vi "Auto Transmission control.vi"(6 "Shift Constants":T1, 7 "In High Gear?":bool, 8 "Time of last recomended shift":u32, 9 "Is Turning?":bool, 10 "Commanded Throttle":dbl, 11 "Avg  encoder speed in fps":dbl) -> (0 "Time of last recomended shift":u32, 3 "should be High Gear?":bool)   [LabVIEW 2013]
uses:
  Shift Constants.ctl
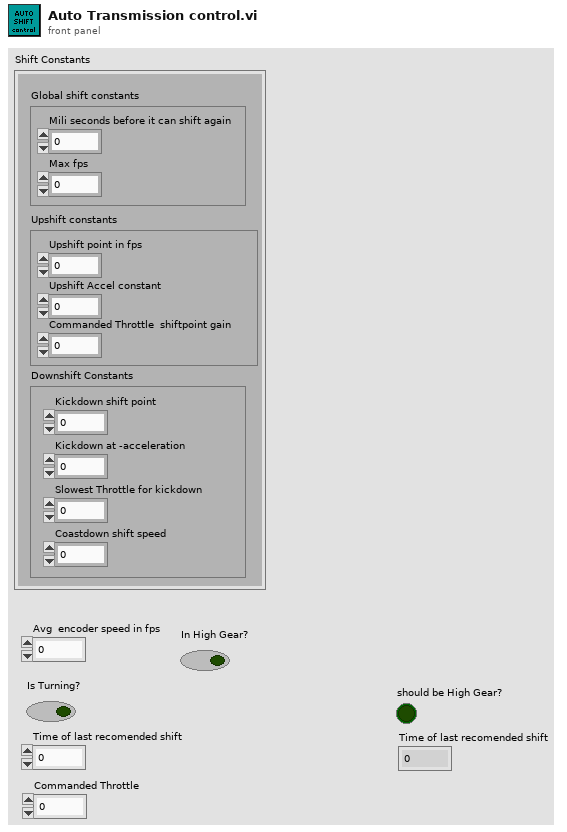
[diagram p1: front panel]
types:
  T1 = typedef "Shift Constants.ctl" = cluster{"Global shift constants":cluster{"Mili seconds before it can shift again":u32, "Max fps":dbl}, "Upshift constants":cluster{"Upshift point in fps":dbl, "Upshift Accel constant":dbl, "Commanded Throttle  shiftpoint gain":dbl}, "Downshift Constants":cluster{"Kickdown shift point":dbl, "Kickdown at -acceleration":dbl, "Slowest Throttle for kickdown":dbl, "Coastdown shift speed":dbl}}
  T2 = cluster{"Mili seconds before it can shift again":u32, "Max fps":dbl}
  T3 = cluster{"Upshift point in fps":dbl, "Upshift Accel constant":dbl, "Commanded Throttle  shiftpoint gain":dbl}
  T4 = cluster{"Kickdown shift point":dbl, "Kickdown at -acceleration":dbl, "Slowest Throttle for kickdown":dbl, "Coastdown shift speed":dbl}
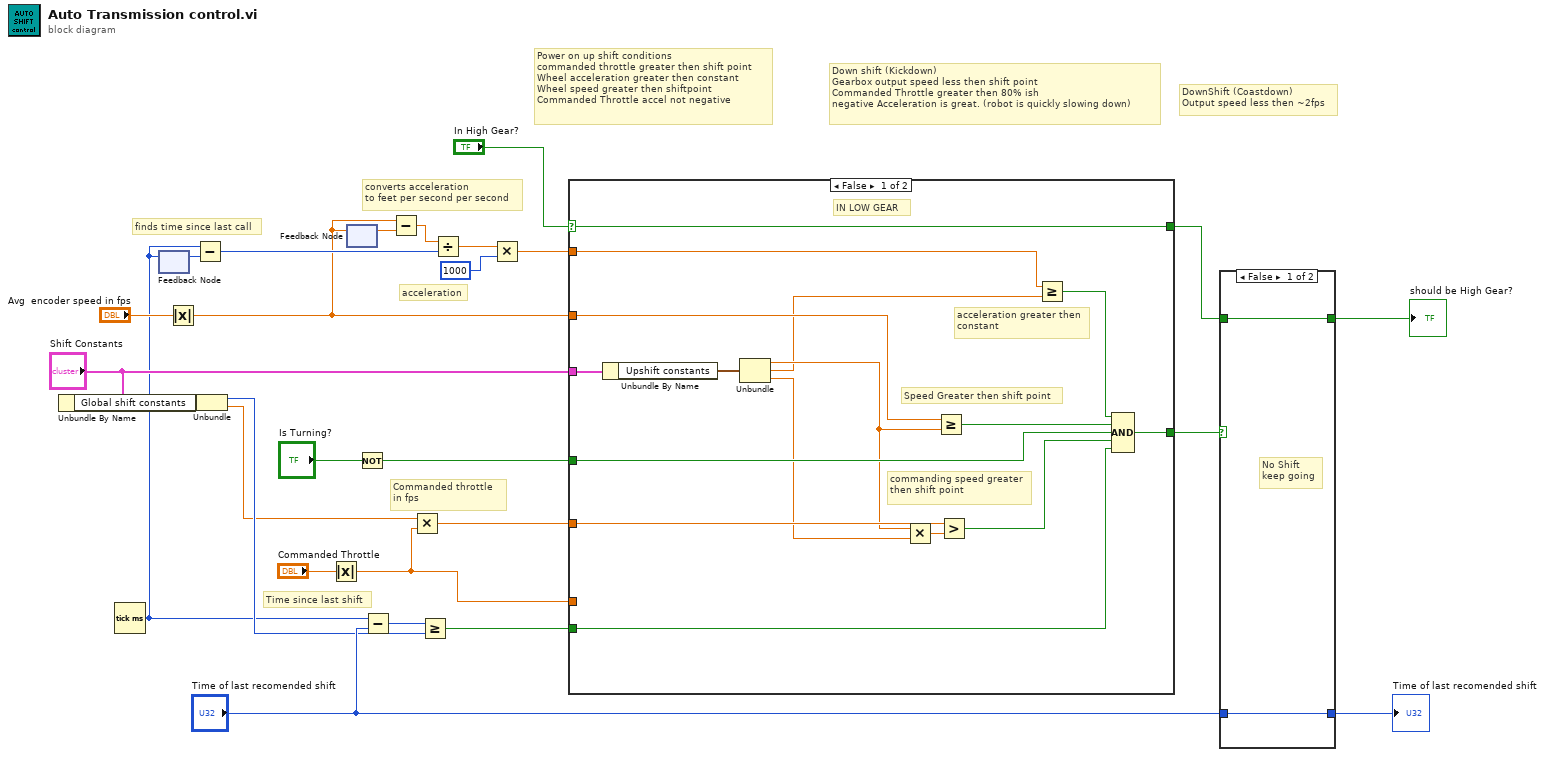
[diagram p0: block diagram]
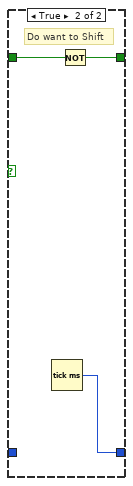
[diagram p2: hidden frame]
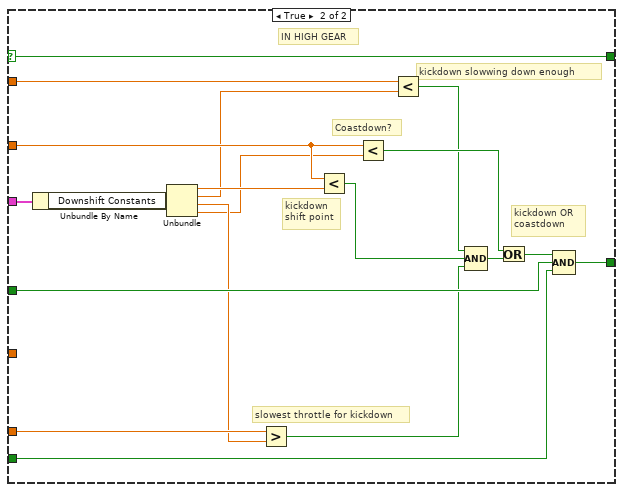
[diagram p3: hidden frame]
diagram:
  # "converts acceleration\nto feet per second per second"
  # "finds time since last call"
  # "DownShift (Coastdown)\nOutput speed less then ~2fps"
  # "Down shift (Kickdown)\nGearbox output speed less then shift point\nCommanded Throttle greater then 80% ish\nnegative Acceleration is great. (robot is quickly slowing down)"
  # "Commanded throttle\nin fps"
  # "Power on up shift conditions\ncommanded throttle greater then shift point\nWheel acceleration greater then constant\nWheel speed greater then shiftpoint\nCommanded Throttle accel not negative"
  # "acceleration"
  # "Time since last shift"
  n1 = Unbundle By Name("Shift Constants") -> ("Global shift constants"=w11:T2)
  n2 = Tick Count (ms)() -> (millisecond timer value=w8:u32)
  n3 = feedback-in #1(w8) -> ()
  n4 = feedback #1() -> (w7:u32)  [unwired: 1 in]
  n5 = Absolute Value(x="Avg  encoder speed in fps") -> (abs(x)=w4:dbl)
  n6 = Subtract(x=w8, y=w7) -> (x-y=w5:u32)
  n7 = Unbundle(w11) -> ("Mili seconds before it can shift again"=w10:u32, "Max fps"=w9:dbl)
  n8 = Absolute Value(x="Commanded Throttle") -> (abs(x)=w13:dbl)
  n9 = feedback #2() -> (w15:dbl)  [unwired: 1 in]
  n10 = feedback-in #2(w4) -> ()
  n11 = Not(x="Is Turning?") -> (.not. x?=w25:bool)
  n12 = Subtract(x=w8, y="Time of last recomended shift") -> (x-y=w19:u32)
  n13 = Subtract(x=w4, y=w15) -> (x-y=w6:dbl)
  n14 = Multiply(x=w9, y=w13) -> (x*y=w14:dbl)
  n15 = Greater Or Equal?(x=w19, y=w10) -> (x >= y?=w18:bool)
  n16 = Divide(x=w6, y=w5) -> (x/y=w2:dbl)
  n17 = Multiply(x=w2, y=i16 1000) -> (x*y=w3:dbl)
  n18 = case shown="False" "In High Gear?" {
    selector: "In High Gear?" -> [w43 w62]
    tunnel: w25 -> [w37 w60]
    tunnel: [w43 w62] -> w23
    tunnel: [w42 w59] -> w24
    tunnel: w18 -> [w33 w61]
    tunnel: w14 -> [w41 _]
    tunnel: w4 -> [w36 w55]
    tunnel: w3 -> [w34 w54]
    tunnel: w13 -> [_ w56]
    tunnel: "Shift Constants" -> [w32 w49]
    frame False {
      # "acceleration greater then\nconstant"
      # "Speed Greater then shift point"
      # "commanding speed greater then shift point"
      # "IN LOW GEAR"
      n19 = Unbundle By Name(w32) -> ("Upshift constants"=w31:T3)
      n20 = Unbundle(w31) -> ("Upshift point in fps"=w30:dbl, "Upshift Accel constant"=w29:dbl, "Commanded Throttle  shiftpoint gain"=w28:dbl)
      n21 = Multiply(x=w30, y=w28) -> (x*y=w40:dbl)
      n22 = Greater Or Equal?(x=w36, y=w30) -> (x >= y?=w38:bool)
      n23 = Greater?(x=w41, y=w40) -> (0:w39:bool)
      n24 = Greater Or Equal?(x=w34, y=w29) -> (x >= y?=w35:bool)
      n25 = Compound Arithmetic op=AND(w35, w38, w37, w39, w33) -> (w42:bool)
    }
    frame True {
      # "kickdown slowwing down enough"
      # "kickdown OR\ncoastdown"
      # "slowest throttle for kickdown"
      # "kickdown\nshift point"
      # "Coastdown?"
      # "IN HIGH GEAR"
      n26 = Unbundle By Name(w49) -> ("Downshift Constants"=w48:T4)
      n27 = Unbundle(w48) -> ("Kickdown shift point"=w47:dbl, "Kickdown at -acceleration"=w46:dbl, "Slowest Throttle for kickdown"=w45:dbl, "Coastdown shift speed"=w44:dbl)
      n28 = Greater?(x=w56, y=w45) -> (0:w51:bool)
      n29 = Less?(x=w55, y=w47) -> (x < y?=w52:bool)
      n30 = Less?(x=w55, y=w44) -> (x < y?=w57:bool)
      n31 = Less?(x=w54, y=w46) -> (x < y?=w53:bool)
      n32 = Compound Arithmetic op=AND(w53, w52, w51) -> (w50:bool)
      n33 = Or(x=w57, y=w50) -> (x .or. y?=w58:bool)
      n34 = Compound Arithmetic op=AND(w58, w60, w61) -> (w59:bool)
    }
  }
  n35 = case shown="False" w24 {
    tunnel: w23 -> [w63 w67]
    tunnel: [w63 w66] -> w22
    tunnel: [w64 w65] -> w21
    tunnel: "Time of last recomended shift" -> [w64 _]
    frame False {
      # "No Shift\nkeep going"
    }
    frame True {
      # "Do want to Shift"
      n36 = Tick Count (ms)() -> (millisecond timer value=w65:u32)
      n37 = Not(x=w67) -> (.not. x?=w66:bool)
    }
  }
  "should be High Gear?" <- w22
  "Time of last recomended shift" <- w21
